vi "CspecCH4_2024.vi"(0 "Temperature [K]":dbl=293.15 format="%.4g") -> (1 "rel. unc. Cp0/R CH":dbl=0.001 format="%.2e", 2 "Cp0/R CH4":dbl=4.272848820630882 format="%.5g", 3 "Cp0 [J / Kmol]":dbl=35.52644171458958, 4 "Cv0 [J / Kmol]":dbl=27.21197911458958, 5 "Gamma0":dbl=1.3055442077545267)   [LabVIEW 2016]
panel:
  out "abs unc Cp0/R N2":dbl=0.008545697641261764 format="%#.4g"
  in  "rel. unc. Cp0/R CH4":dbl=0.001 format="%.2e"
  # "Methane - Setzmann & Wagner J. Phys. Chem. Ref. Data 1991 - Eq. (3.8)"
  # "Calculated using Eq. 3.8 with coefficients from Table 27 in EoS methane Setzmann & Wagner [18] supposed valid between 60 K and 3000 K.\nThis equation is based on spectroscopic data and calculations by Mc-Dowell and Kruse. Deviations from this source estimate 0.07% at maximum.\nRelative uncertainty fixed here to be 0.1% over the whole temperature range. These reference sources differ by  those of Zuckerwar by -0.41% at 273.16 K"
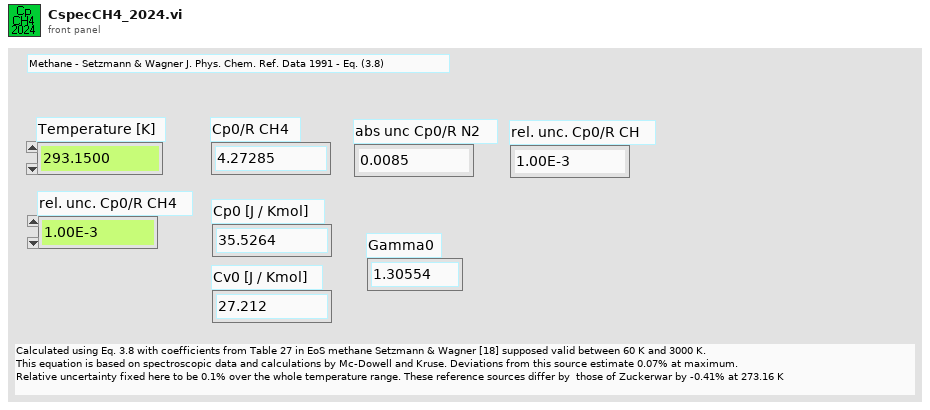
[diagram p1: front panel]
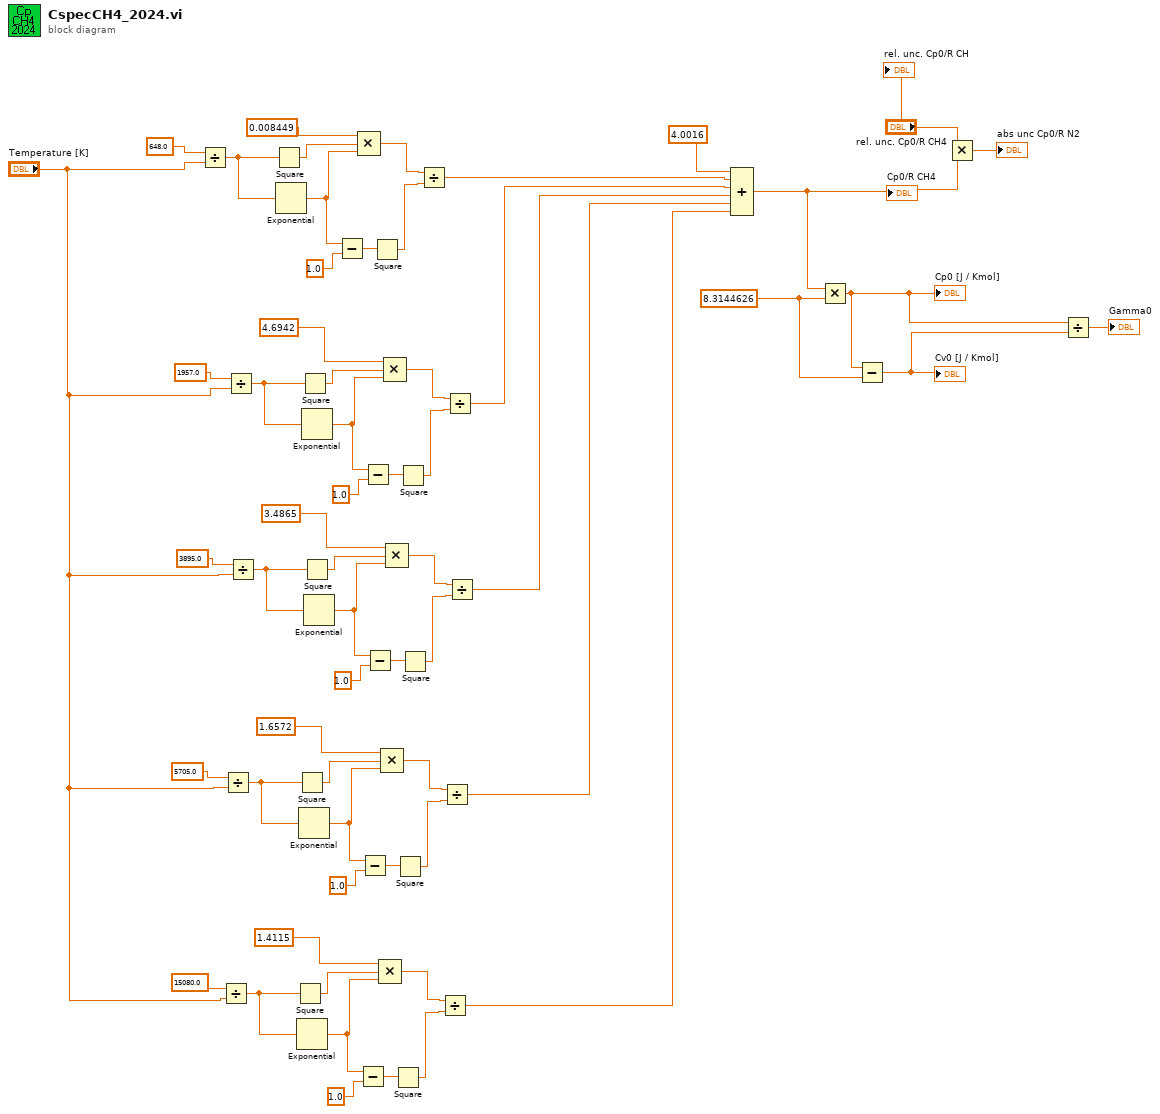
[diagram p0: block diagram]
diagram:
  w7 = 8.3144626
  n1 = Divide(x=648.0, y="Temperature [K]") -> (x/y=w55:dbl)
  n2 = Divide(x=15080.0, y="Temperature [K]") -> (x/y=w20:dbl)
  n3 = Divide(x=5705.0, y="Temperature [K]") -> (x/y=w29:dbl)
  n4 = Divide(x=1957.0, y="Temperature [K]") -> (x/y=w46:dbl)
  n5 = Divide(x=3895.0, y="Temperature [K]") -> (x/y=w37:dbl)
  n6 = Square(x=w55) -> (x^2=w56:dbl)
  n7 = Exponential(1:w55) -> (0:w54:dbl)
  n8 = Square(x=w20) -> (x^2=w21:dbl)
  n9 = Square(x=w29) -> (x^2=w30:dbl)
  n10 = Exponential(1:w20) -> (0:w19:dbl)
  n11 = Exponential(1:w29) -> (0:w28:dbl)
  n12 = Square(x=w46) -> (x^2=w47:dbl)
  n13 = Exponential(1:w46) -> (0:w45:dbl)
  n14 = Square(x=w37) -> (x^2=w38:dbl)
  n15 = Exponential(1:w37) -> (0:w36:dbl)
  n16 = Subtract(x=w54, y=1.0) -> (x-y=w52:dbl)
  n17 = Compound Arithmetic op=MULTIPLY(0.008449, w56, w54) -> (w51:dbl)
  n18 = Subtract(x=w19, y=1.0) -> (x-y=w17:dbl)
  n19 = Subtract(x=w28, y=1.0) -> (x-y=w26:dbl)
  n20 = Subtract(x=w45, y=1.0) -> (x-y=w43:dbl)
  n21 = Subtract(x=w36, y=1.0) -> (x-y=w34:dbl)
  n22 = Square(x=w52) -> (x^2=w50:dbl)
  n23 = Compound Arithmetic op=MULTIPLY(1.4115, w21, w19) -> (w16:dbl)
  n24 = Compound Arithmetic op=MULTIPLY(1.6572, w30, w28) -> (w25:dbl)
  n25 = Compound Arithmetic op=MULTIPLY(4.6942, w47, w45) -> (w42:dbl)
  n26 = Compound Arithmetic op=MULTIPLY(3.4865, w38, w36) -> (w33:dbl)
  n27 = Square(x=w17) -> (x^2=w15:dbl)
  n28 = Square(x=w26) -> (x^2=w24:dbl)
  n29 = Square(x=w43) -> (x^2=w41:dbl)
  n30 = Square(x=w34) -> (x^2=w32:dbl)
  n31 = Divide(x=w51, y=w50) -> (x/y=w12:dbl)
  n32 = Divide(x=w16, y=w15) -> (x/y=w8:dbl)
  n33 = Divide(x=w25, y=w24) -> (x/y=w9:dbl)
  n34 = Divide(x=w42, y=w41) -> (x/y=w11:dbl)
  n35 = Divide(x=w33, y=w32) -> (x/y=w10:dbl)
  n36 = Compound Arithmetic op=ADD(4.0016, w12, w11, w10, w9, w8) -> (w2:dbl)
  "Cp0/R CH4" <- w2
  n37 = Multiply(x=w2, y=w7) -> (x*y=w6:dbl)
  "Cp0 [J / Kmol]" <- w6
  n38 = Subtract(x=w6, y=w7) -> (x-y=w5:dbl)
  "Cv0 [J / Kmol]" <- w5
  n39 = Multiply(x="rel. unc. Cp0/R CH4", y=w2) -> (x*y=→"abs unc Cp0/R N2":dbl)
  n40 = Divide(x=w6, y=w5) -> (x/y=→"Gamma0":dbl)
  "rel. unc. Cp0/R CH" <- "rel. unc. Cp0/R CH4"
